vi "Configure Volume.vi"(7 "Save":bool, 8 "error in (no error)":errorcluster, 9 "NumReps":i32, 10 "Scan Settings":T1, 11 "AODAcq in":refnum<class "AODAcq.lvclass">) -> (0 "error out":errorcluster, 3 "AODAcq out":refnum<class "AODAcq.lvclass">)   [LabVIEW 2014, in "AODAcq.lvclass"]
uses:
  AODAcq.lvclass
  AODAcq.lvclass/AODAcq.ctl
  <vilib>/Utility/error.llb/Error Cluster From Error Code.vi
  C:/Program Files (x86)/National Instruments/LabVIEW 2014/Targets/NI/FPGA/StockFPGA_IntfPrivate/ScriptTemplates/StockFPGA_PlugInRead32.vi
  <vilib>/rvi/errors/niLvFpgaAdjustHostInterfaceError.vi
  <vilib>/rvi/interface/nirviReadWriteControl/nirviReadWriteControl.xnode
  FPGA_Control/AODRef.ctl
  FPGA Bitfiles/AodScanner_FPGATarget_AODControl(FPGA)_TyJc9yYmyGA.lvbitx
  HDF5Tools/LabView/HDF5Tools.lvlib
  NiFpgaLv.dll
  <vilib>/FPGAPlugInAG/PXIe-7965R/niLvFpga_Read32_PXIe-7965R.vi
  <vilib>/rvi/interface/nirviReadWriteControl/niFpgaRWControlAccessTimeoutTemplate.vi
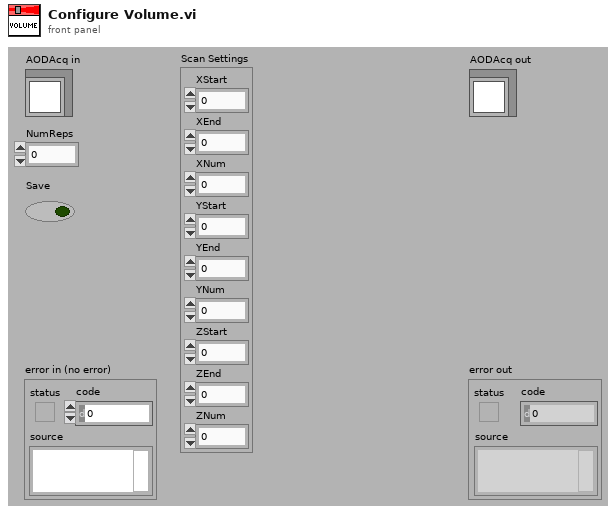
[diagram p1: front panel]
types:
  T1 = cluster{"XStart":i32, "XEnd":i32, "XNum":i32, "YStart":i32, "YEnd":i32, "YNum":i32, "ZStart":i32, "ZEnd":i32, "ZNum":i32}
  T2 = typedef "AODRef.ctl" = refnum<k20>
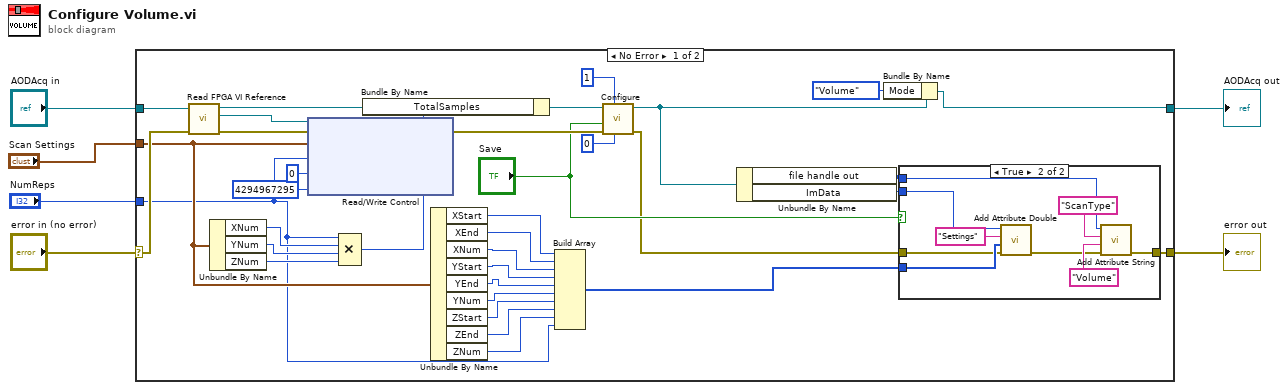
[diagram p0: block diagram]
diagram:
  n1 = case shown="No Error" "error in (no error)" {
    selector: "error in (no error)" -> [w36 w53]
    tunnel: [w8 w53] -> w5
    tunnel: [w16 w52] -> w3
    tunnel: "AODAcq in" -> [w41 w52]
    tunnel: "Scan Settings" -> [w21 _]
    tunnel: "NumReps" -> [w19 _]
    frame No Error {
      n2 = call-dynamic "Read FPGA VI Reference.vi"("error in (no error)"=w36, "AODAcq in"=w41) -> ("error out"=w39:errorcluster, "FPGA VI Reference"=w40:T2, "AODAcq out"=w31:refnum<class "AODAcq.lvclass">)  [unwired: 7 in]
      n3 = Unbundle By Name(w21) -> ("XNum"=w33:i32, "YNum"=w34:i32, "ZNum"=w35:i32)
      n4 = xnode "Read/Write Control"("FPGA VI Reference In"=w40, "error in"=w39, "Scan.VolumeSettings"=w21, "Scan.NumReps"=w19, "Scan.NumMotionPoints"=u32 0, "Scan.Motion Increment"=u32 4294967295) -> ("error out"=w37:errorcluster)  [unwired: 1 out]
      n5 = Compound Arithmetic op=MULTIPLY(w19, w33, w34, w35) -> (w32:i32)
      n6 = Bundle By Name(cluster=w31, "TotalSamples"=w32) -> (w30:refnum<class "AODAcq.lvclass">)
      n7 = Unbundle By Name(w21) -> ("XStart"=w20:i32, "XEnd"=w22:i32, "XNum"=w23:i32, "YStart"=w24:i32, "YEnd"=w25:i32, "YNum"=w26:i32, "ZStart"=w27:i32, "ZEnd"=w28:i32, "ZNum"=w29:i32)
      n8 = Build Array(w20, w22, w23, w24, w25, w26, w27, w28, w29, w19) -> (w11:i32[])
      n9 = call-dynamic "Configure.vi"("GridSize"=u32 0, "Mode"=u32 1, "error in (no error)"=w37, "Save"="Save", "AODAcq in"=w30) -> ("error out"=w9:errorcluster, "AODAcq out"=w18:refnum<class "AODAcq.lvclass">)  [unwired: 5 in]
      n10 = Unbundle By Name(w18) -> ("file handle out"=w7:i32, "ImData"=w12:i32)
      n11 = Bundle By Name(cluster=w18, "Mode"=enum16{"Idle", "Points", "Volume"}."Volume") -> (w16:refnum<class "AODAcq.lvclass">)
      n12 = case shown="True" "Save" {
        tunnel: w12 -> [_ w51]
        tunnel: w11 -> [_ w49]
        tunnel: w9 -> [w42 w48]
        tunnel: [w42 w45] -> w8
        tunnel: w7 -> [_ w43]
        frame False {
        }
        frame True {
          n13 = call "Add Attribute Double.vi"("error in (no error)"=w48, "data"=w49, "Attribute name"="Settings", "loc_id"=w51) -> ("error out"=w44:errorcluster)  [unwired: 6 in, 1 out]
          n14 = call "Add Attribute String.vi"("error in (no error)"=w44, "Attribute data"="Volume", "Attribute name"="ScanType", "loc_id"=w43) -> ("error out"=w45:errorcluster)  [unwired: 6 in, 1 out]
        }
      }
    }
    frame Error {
    }
  }
  "error out" <- w5
  "AODAcq out" <- w3
